vi "Wait for Dashboard.vi"(8 "Timeout (s)":dbl=1.0, 11 "Count":i32) -> (2 "Timeout":bool)   [LabVIEW 2017]
doc: "This VI allows portions of your robot code to wait until Network Table connection(s) have been established and initialized. You can specify how many connections and how log to wait in seconds. The output value indicates whether the VI completed because of a timeout."
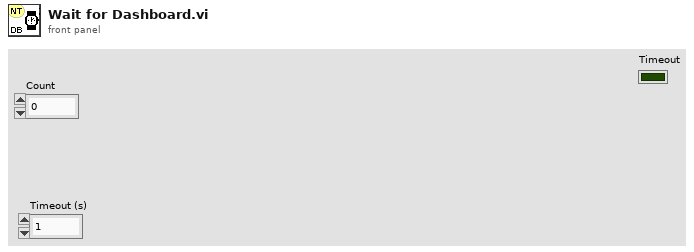
[diagram p1: front panel]
types:
  T1 = enum16{"Add Cnx", "Remove Cnx", "Retrieve List", "Cnx Inited"}
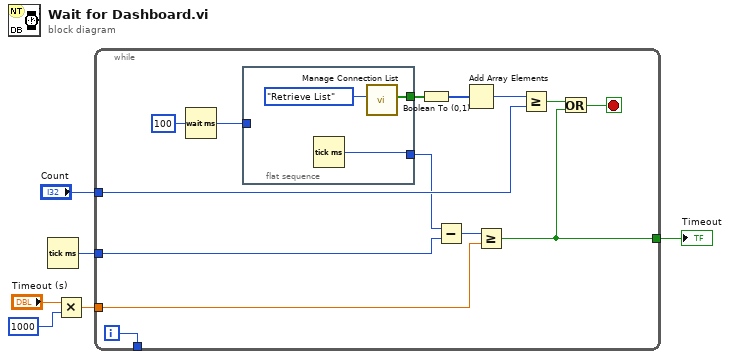
[diagram p0: block diagram]
diagram:
  n1 = Tick Count (ms)() -> (millisecond timer value=w5:u32)
  n2 = Multiply(x="Timeout (s)", y=1000) -> (x*y=w2:dbl)
  n3 = while {
    tunnel: "Count" -> [w18]
    tunnel: w5 -> [w16]
    tunnel: w2 -> [w13]
    tunnel: [w8] -> w1
    tunnel: [w7] -> _
    i -> [w7]
    stop <- w12 stop-if-true
    n4 = Wait (ms)(milliseconds to wait=u32 100) -> (millisecond timer value=w11:u32)
    n5 = flat-sequence {
      tunnel: [w22] -> w20
      tunnel: w11 -> [_]
      tunnel: [w21] -> w9
      frame #0 {
        n6 = Tick Count (ms)() -> (millisecond timer value=w21:u32)
        n7 = call <vilib>:"Manage Connection List.vi"("Operation"=T1."Retrieve List") -> ("Inited"=w22:bool[])  [unwired: 8 in, 2 out]
      }
    }
    n8 = Boolean To (0,1)(Boolean=w20) -> (0, 1=w19:i16[])
    n9 = Subtract(x=w9, y=w16) -> (x-y=w14:u32)
    n10 = Add Array Elements(numeric array=w19) -> (sum=w17:i16)
    n11 = Greater Or Equal?(x=w14, y=w13) -> (x >= y?=w8:bool)
    n12 = Greater Or Equal?(x=w17, y=w18) -> (x >= y?=w15:bool)
    n13 = Or(x=w15, y=w8) -> (x .or. y?=w12:bool)
  }
  "Timeout" <- w1
